vi "Variant To LVType.vi"(8 "error in (no error)":errorcluster, 11 "Variant":variant) -> (0 "error out":errorcluster, 3 "LVType":refnum<class "LVType.lvclass">)   [LabVIEW 2020, in "LVDataTypes.lvlib"]
uses:
  <vilib>/AppBuilder/Engine/WebServiceDescription/LVDataTypes/LVDataTypes.lvlib
  <vilib>/AppBuilder/Engine/WebServiceDescription/LVDataTypes/TypeCode.ctl
  <vilib>/AppBuilder/Engine/WebServiceDescription/LVDataTypes/LVType/LVType.lvclass
  <vilib>/Utility/VariantDataType/Type.ctl
  <vilib>/AppBuilder/Engine/WebServiceDescription/LVDataTypes/LVEnum/LVEnum.lvclass
  e:/builds/penguin/labview/branches/2020/dev/dist/vi.lib/AppBuilder/Engine/WebServiceDescription/LVDataTypes/LVType/LVType.lvclass
  <vilib>/AppBuilder/Engine/WebServiceDescription/LVDataTypes/LVArrayType/LVArrayType.lvclass
  <vilib>/AppBuilder/Engine/WebServiceDescription/LVDataTypes/LVAnalogWaveformType/LVAnalogWaveformType.lvclass
  <vilib>/AppBuilder/Engine/WebServiceDescription/LVDataTypes/LVClusterType/LVClusterType.lvclass
  <vilib>/Utility/VariantDataType/VariantType.lvlib
panel:
  in  "Type Enum":T1
  in  "TypeMap":T2[](array[typedef])=[enum."Undefined", enum."Void", enum."Byte", enum."Word", enum."Long", enum."Quad", enum."Unsigned Byte", enum."Unsigned Word", enum."Unsigned Long", enum."Unsigned Quad", enum."Single", enum."Double", enum."Extended", enum."Complex Single", enum."Complex Double", enum."Complex Extended", enum."Unsigned Byte", enum."Unsigned Word", enum."Unsigned Long", enum."Unsigned Quad", enum."Single", enum."Double", enum."Extended", enum."Complex Single", enum."Complex Double", enum."Complex Extended", enum."Boolean", enum."String", enum."Path", enum."Undefined", enum."Undefined", enum."Array", enum."Cluster", enum."Undefined", enum."Undefined", enum."AnalogWaveform", enum."Time Stamp", enum."DigitalWaveform", enum."Undefined", enum."Undefined", enum."Undefined", enum."Undefined", enum."Undefined", enum."Undefined", enum."Undefined", enum."Undefined"]
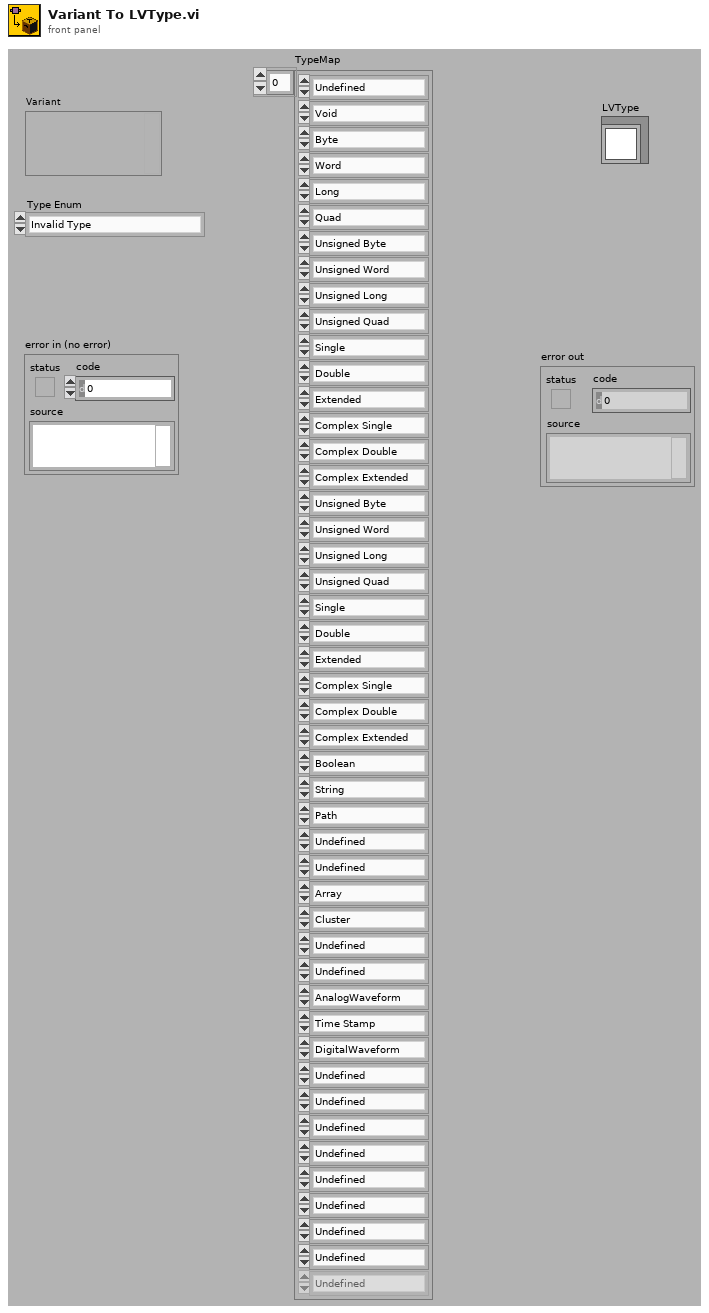
[diagram p1: front panel]
types:
  T1 = typedef "VariantType.lvlib/Type.ctl" = enum8{"Invalid Type", "Void", "I8", "I16", "I32", "I64", "U8", "U16", "U32", "U64", "Single Float", "Double Float", "Extended Float", "Single Complex", "Double Complex", "Extended Complex", "Enum U8", "Enum U16", "Enum U32", "Enum U64", "Single Float With Unit", "Double Float With Unit", "Extended Float With Unit", "Single Complex with Unit", "Double Complex with Unit", "Extended Complex with Unit", "Boolean", "String", "Path", "Picture", "Tag", "Array", "Cluster", "Variant", "LV Variant", "Waveform", "Timestamp", "Digital Waveform", "Digital Data", "ExpressData", "Refnum", "External Data", "VI", "Poly VI", "LabVIEW Class Instance", "Fixed Point"}
  T2 = typedef "LVDataTypes.lvlib/TypeCode.ctl" = enum16{"Undefined", "Byte", "Unsigned Byte", "Word", "Unsigned Word", "Long", "Unsigned Long", "Quad", "Unsigned Quad", "Single", "Double", "Extended", "Enum", "Boolean", "String", "Path", "Array", "Cluster", "AnalogWaveform", "DigitalWaveform", "Time Stamp", "Void", "Complex Single", "Complex Double", "Complex Extended"}
  T3 = typedef "VariantType.lvlib/MemoryInfo.ctl" = cluster{"Type":T4, "Size":u32}
  T4 = typedef "VariantType.lvlib/MemoryType.ctl" = enum16{"Variable", "Fixed", "Bounded"}
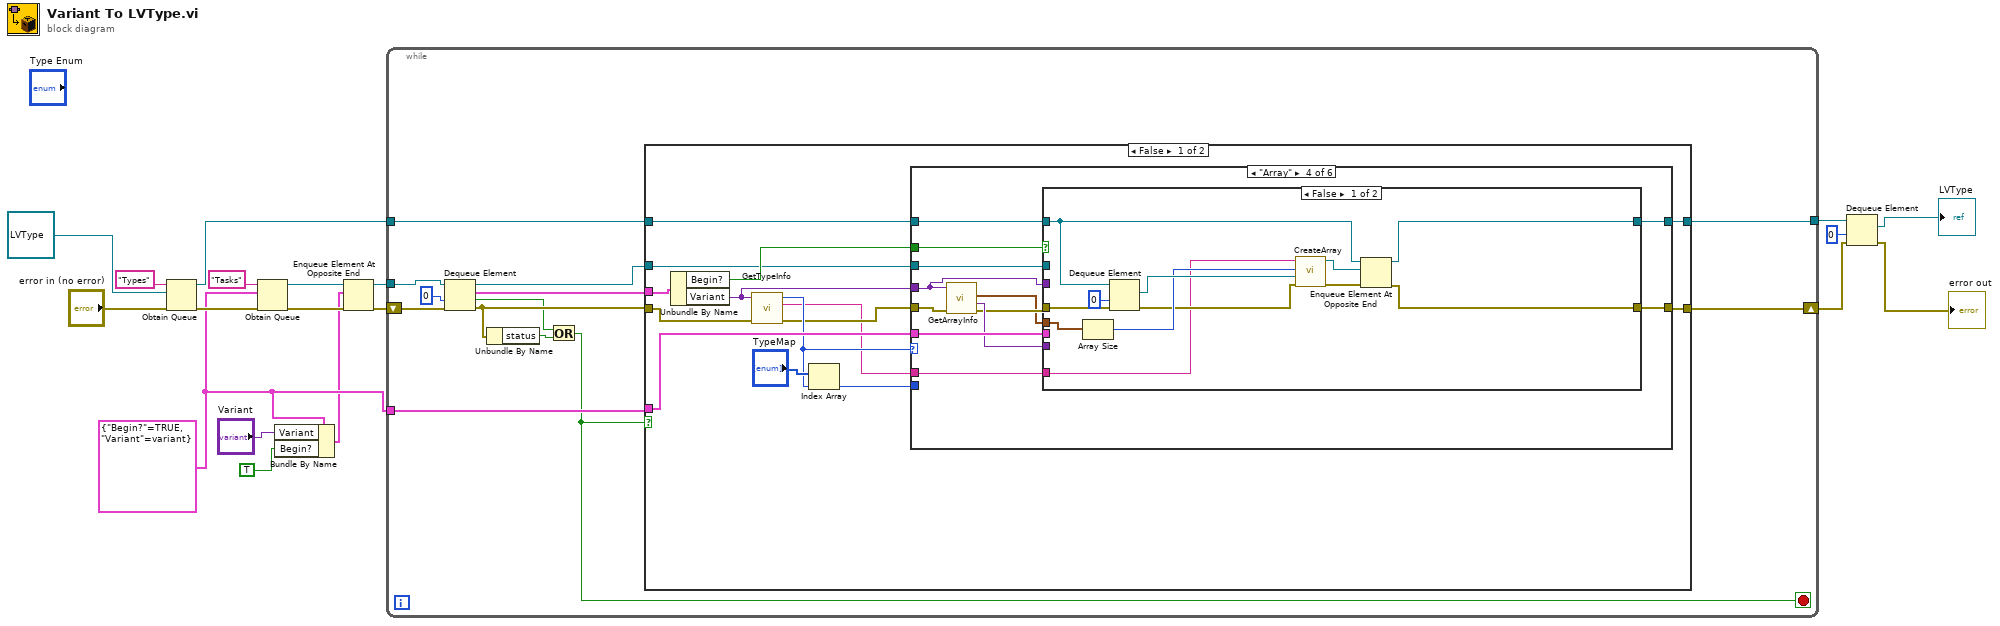
[diagram p0: block diagram]
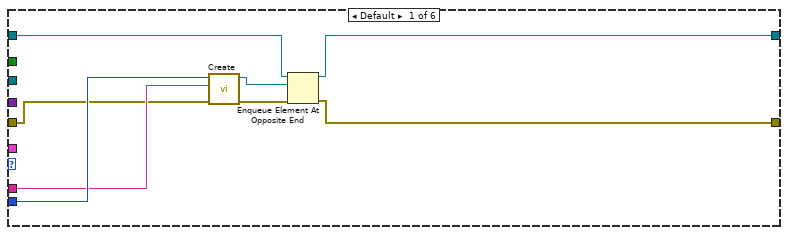
[diagram p2: hidden frame]
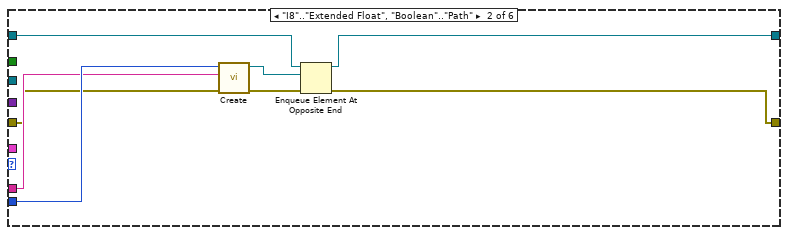
[diagram p3: hidden frame]
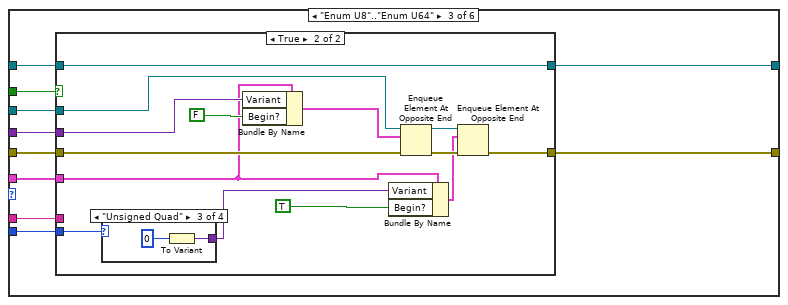
[diagram p4: hidden frame]
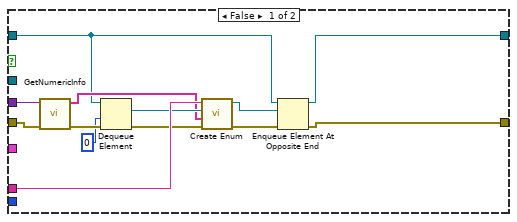
[diagram p5: hidden frame]
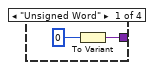
[diagram p6: hidden frame]
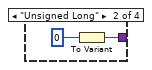
[diagram p7: hidden frame]
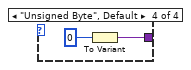
[diagram p8: hidden frame]
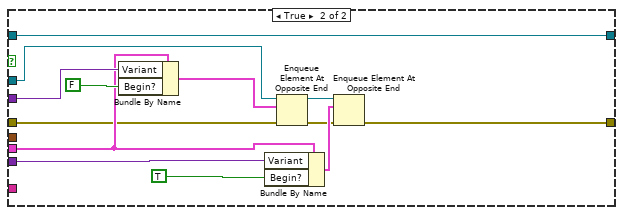
[diagram p9: hidden frame]
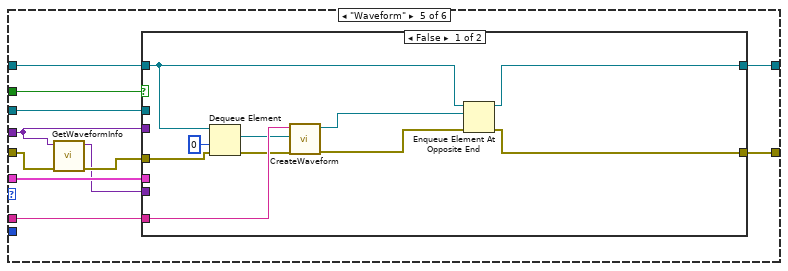
[diagram p10: hidden frame]
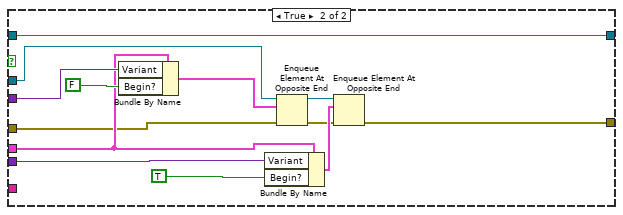
[diagram p11: hidden frame]
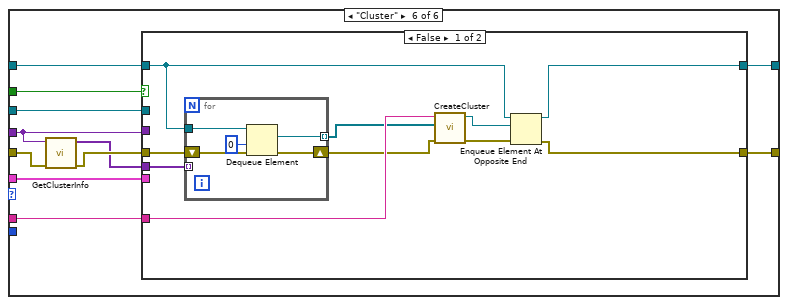
[diagram p12: hidden frame]
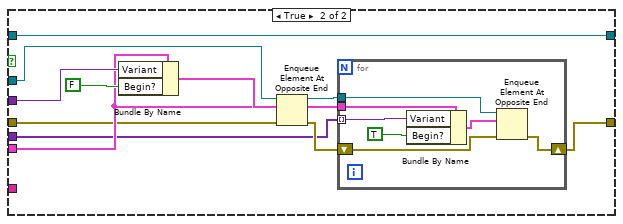
[diagram p13: hidden frame]
diagram:
  w15 = cluster{"Begin?":bool, "Variant":variant} {"Begin?"=TRUE, "Variant"=variant}
  n1 = Obtain Queue(name (unnamed)="Types", element data type=refnum<class "LVType.lvclass"> refnum ("LVDataTypes.lvlib:LVType.lvclass"), error in (no error)="error in (no error)") -> (queue out=w19:refnum<queue>, error out=w18:errorcluster)  [unwired: 2 in, 1 out]
  n2 = Obtain Queue(name (unnamed)="Tasks", element data type=w15, error in (no error)=w18) -> (queue out=w10:refnum<queue>, error out=w12:errorcluster)  [unwired: 2 in, 1 out]
  n3 = Bundle By Name(cluster=w15, "Variant"="Variant", "Begin?"=TRUE) -> (w11:cluster{"Begin?":bool, "Variant":variant})
  n4 = Enqueue Element At Opposite End(queue=w10, element=w11, error in (no error)=w12) -> (queue out=w14:refnum<queue>, error out=w13:errorcluster)  [unwired: 2 out]
  n5 = while {
    tunnel: w14 -> [w32]
    shift-right: [w26] -> w4
    shift-left: w13 -> [w31]
    tunnel: w15 -> [w27]
    tunnel: w19 -> [w25]
    tunnel: [w24] -> w6
    stop <- w20 stop-if-true
    n6 = Dequeue Element(queue=w32, timeout in ms (-1)=0, error in (no error)=w31) -> (queue out=w28:refnum<queue>, element=w29:cluster{"Begin?":bool, "Variant":variant}, timed out?=w21:bool, error out=w23:errorcluster)
    n7 = Unbundle By Name(w23) -> ("status"=w22:bool)
    n8 = Or(x=w21, y=w22) -> (x .or. y?=w20:bool)
    n9 = case shown="False" w20 {
      tunnel: w29 -> [w46 _]
      tunnel: w23 -> [w40 w224]
      tunnel: w28 -> [w44 _]
      tunnel: w27 -> [w43 _]
      tunnel: [w42 w224] -> w26
      tunnel: w25 -> [w41 w223]
      tunnel: [w33 w223] -> w24
      frame False {
        n10 = Unbundle By Name(w46) -> ("Begin?"=w45:bool, "Variant"=w36:variant)
        n11 = call <vilib>:"GetTypeInfo.vi"("error in (no error)"=w40, "Variant"=w36) -> ("error out"=w37:errorcluster, "Name"=w35:string, "Type Enum"=w38:T1)  [unwired: 7 out]
        n12 = Index Array(array="TypeMap", index=w38) -> (element=w34:T2)
        n13 = case shown="\"Array\"" w38 {
          tunnel: w37 -> [w52 w60 w67 w114 w147 w181]
          tunnel: w45 -> [_ _ w69 w119 w155 w189]
          tunnel: w44 -> [_ _ w70 w118 w154 w188]
          tunnel: w43 -> [_ _ w66 w117 w153 w187]
          tunnel: [w47 w58 w63 w116 w152 w186] -> w42
          tunnel: w41 -> [w50 w57 w72 w115 w151 w185]
          tunnel: w36 -> [_ _ w68 w113 w148 w182]
          tunnel: w35 -> [w53 w61 w64 w109 w150 w184]
          tunnel: w34 -> [w54 w62 w65 _ _ _]
          tunnel: [w48 w55 w71 w108 w149 w183] -> w33
          frame Default {
            n14 = call <vilib>:"Create.vi"("error in (no error)"=w52, "ID"=w53, "Type"=w54) -> ("error out"=w51:errorcluster, "LVType out"=w49:refnum<class "LVType.lvclass">)  [unwired: 7 out]
            n15 = Enqueue Element At Opposite End(queue=w50, element=w49, error in (no error)=w51) -> (queue out=w48:refnum<queue>, error out=w47:errorcluster)  [unwired: 2 out]
          }
          frame "I8".."Extended Float", "Boolean".."Path" {
            n16 = call <vilib>:"Create.vi"("error in (no error)"=w60, "ID"=w61, "Type"=w62) -> ("error out"=w59:errorcluster, "LVType out"=w56:refnum<class "LVType.lvclass">)  [unwired: 7 out]
            n17 = Enqueue Element At Opposite End(queue=w57, element=w56, error in (no error)=w59) -> (queue out=w55:refnum<queue>, error out=w58:errorcluster)  [unwired: 2 out]
          }
          frame "Enum U8".."Enum U64" {
            n18 = case shown="True" w69 {
              tunnel: w72 -> [w77 w93]
              tunnel: [w73 w93] -> w71
              tunnel: w70 -> [_ w92]
              tunnel: w68 -> [w85 w91]
              tunnel: w67 -> [w84 w90]
              tunnel: w66 -> [_ w89]
              tunnel: w65 -> [_ w88]
              tunnel: w64 -> [w81 _]
              tunnel: [w74 w86] -> w63
              frame False {
                n19 = call <vilib>:"GetNumericInfo.vi"("error in (no error)"=w84, "Variant"=w85) -> ("error out"=w83:errorcluster, "EnumNames"=w79:string[])  [unwired: 8 out]
                n20 = Dequeue Element(queue=w77, timeout in ms (-1)=0, error in (no error)=w83) -> (element=w80:refnum<class "LVType.lvclass">, error out=w78:errorcluster)  [unwired: 2 out]
                n21 = call <vilib>:"Create Enum.vi"("error in (no error)"=w78, "Choices"=w79, "BaseType"=w80, "ID"=w81) -> ("error out"=w76:errorcluster, "LVEnum out"=w75:refnum<class "LVEnum.lvclass">)  [unwired: 6 out]
                n22 = Enqueue Element At Opposite End(queue=w77, element=w75, error in (no error)=w76) -> (queue out=w73:refnum<queue>, error out=w74:errorcluster)  [unwired: 2 out]
              }
              frame True {
                n23 = case shown="\"Unsigned Quad\"" w88 {
                  tunnel: [w100 w102 w104 w106] -> w87
                  frame "Unsigned Word" {
                    n24 = To Variant(anything=u16 0) -> (Variant=w100:variant)
                  }
                  frame "Unsigned Long" {
                    n25 = To Variant(anything=u32 0) -> (Variant=w102:variant)
                  }
                  frame "Unsigned Quad" {
                    n26 = To Variant(anything=u64 0) -> (Variant=w104:variant)
                  }
                  frame "Unsigned Byte", Default {
                    n27 = To Variant(anything=u8 0) -> (Variant=w106:variant)
                  }
                }
                n28 = Bundle By Name(cluster=w89, "Variant"=w91, "Begin?"=FALSE) -> (w95:cluster{"Begin?":bool, "Variant":variant})
                n29 = Bundle By Name(cluster=w89, "Variant"=w87, "Begin?"=TRUE) -> (w97:cluster{"Begin?":bool, "Variant":variant})
                n30 = Enqueue Element At Opposite End(queue=w92, element=w95, error in (no error)=w90) -> (queue out=w99:refnum<queue>, error out=w98:errorcluster)  [unwired: 2 out]
                n31 = Enqueue Element At Opposite End(queue=w99, element=w97, error in (no error)=w98) -> (error out=w86:errorcluster)  [unwired: 3 out]
              }
            }
          }
          frame "Array" {
            n32 = call <vilib>:"GetArrayInfo.vi"("error in (no error)"=w114, "Variant"=w113) -> ("error out"=w111:errorcluster, "ArrayElement"=w112:variant, "Array Lengths"=w110:T3[])  [unwired: 7 out]
            n33 = case shown="False" w119 {
              tunnel: w113 -> [_ w141]
              tunnel: w118 -> [_ w142]
              tunnel: w117 -> [_ w138]
              tunnel: [w122 w135] -> w116
              tunnel: w115 -> [w124 w132]
              tunnel: w111 -> [w131 w133]
              tunnel: w112 -> [_ w134]
              tunnel: w110 -> [w128 _]
              tunnel: w109 -> [w125 _]
              tunnel: [w121 w132] -> w108
              frame False {
                n34 = Array Size(array=w128) -> (size(s)=w127:i32)
                n35 = Dequeue Element(queue=w124, timeout in ms (-1)=0, error in (no error)=w131) -> (element=w129:refnum<class "LVType.lvclass">, error out=w126:errorcluster)  [unwired: 2 out]
                n36 = call <vilib>:"CreateArray.vi"("error in (no error)"=w126, "ChildType"=w129, "Dimension"=w127, "ID"=w125) -> ("error out"=w123:errorcluster, "LVArrayType out"=w120:refnum<class "LVArrayType.lvclass">)  [unwired: 6 out]
                n37 = Enqueue Element At Opposite End(queue=w124, element=w120, error in (no error)=w123) -> (queue out=w121:refnum<queue>, error out=w122:errorcluster)  [unwired: 2 out]
              }
              frame True {
                n38 = Bundle By Name(cluster=w138, "Variant"=w141, "Begin?"=FALSE) -> (w143:cluster{"Begin?":bool, "Variant":variant})
                n39 = Bundle By Name(cluster=w138, "Variant"=w134, "Begin?"=TRUE) -> (w139:cluster{"Begin?":bool, "Variant":variant})
                n40 = Enqueue Element At Opposite End(queue=w142, element=w143, error in (no error)=w133) -> (queue out=w136:refnum<queue>, error out=w137:errorcluster)  [unwired: 2 out]
                n41 = Enqueue Element At Opposite End(queue=w136, element=w139, error in (no error)=w137) -> (error out=w135:errorcluster)  [unwired: 3 out]
              }
            }
          }
          frame "Waveform" {
            n42 = call <vilib>:"GetWaveformInfo.vi"("error in (no error)"=w147, "Variant"=w148) -> ("error out"=w146:errorcluster, "YArrayType"=w145:variant)  [unwired: 8 out]
            n43 = case shown="False" w155 {
              tunnel: w148 -> [_ w175]
              tunnel: w154 -> [_ w176]
              tunnel: w153 -> [_ w172]
              tunnel: [w163 w169] -> w152
              tunnel: w151 -> [w164 w167]
              tunnel: w145 -> [_ w168]
              tunnel: w150 -> [w161 _]
              tunnel: [w162 w167] -> w149
              tunnel: w146 -> [w156 w166]
              frame False {
                n44 = Dequeue Element(queue=w164, timeout in ms (-1)=0, error in (no error)=w156) -> (element=w159:refnum<class "LVType.lvclass">, error out=w160:errorcluster)  [unwired: 2 out]
                n45 = call <vilib>:"CreateWaveform.vi"("error in (no error)"=w160, "YArrayType"=w159, "ID"=w161) -> ("error out"=w158:errorcluster, "LVAnalogWaveformType out"=w157:refnum<class "LVAnalogWaveformType.lvclass">)  [unwired: 7 out]
                n46 = Enqueue Element At Opposite End(queue=w164, element=w157, error in (no error)=w158) -> (queue out=w162:refnum<queue>, error out=w163:errorcluster)  [unwired: 2 out]
              }
              frame True {
                n47 = Bundle By Name(cluster=w172, "Variant"=w175, "Begin?"=FALSE) -> (w177:cluster{"Begin?":bool, "Variant":variant})
                n48 = Bundle By Name(cluster=w172, "Variant"=w168, "Begin?"=TRUE) -> (w173:cluster{"Begin?":bool, "Variant":variant})
                n49 = Enqueue Element At Opposite End(queue=w176, element=w177, error in (no error)=w166) -> (queue out=w170:refnum<queue>, error out=w171:errorcluster)  [unwired: 2 out]
                n50 = Enqueue Element At Opposite End(queue=w170, element=w173, error in (no error)=w171) -> (error out=w169:errorcluster)  [unwired: 3 out]
              }
            }
          }
          frame "Cluster" {
            n51 = call <vilib>:"GetClusterInfo.vi"("error in (no error)"=w181, "Variant"=w182) -> ("error out"=w180:errorcluster, "Cluster Elements"=w179:variant[])  [unwired: 8 out]
            n52 = case shown="False" w189 {
              tunnel: w182 -> [_ w212]
              tunnel: w188 -> [_ w213]
              tunnel: w187 -> [_ w211]
              tunnel: [w191 w206] -> w186
              tunnel: w185 -> [w192 w209]
              tunnel: w180 -> [w199 w210]
              tunnel: w184 -> [w197 _]
              tunnel: [w190 w209] -> w183
              tunnel: w179 -> [w198 w205]
              frame False {
                n53 = for {
                  tunnel: w192 -> [w202]
                  tunnel: w198 -> [_] mode=indexing
                  tunnel: [w201] -> w196 mode=indexing
                  shift-right: [w200] -> w195
                  shift-left: w199 -> [w204]
                  n54 = Dequeue Element(queue=w202, timeout in ms (-1)=0, error in (no error)=w204) -> (element=w201:refnum<class "LVType.lvclass">, error out=w200:errorcluster)  [unwired: 2 out]
                }
                n55 = call <vilib>:"CreateCluster.vi"("error in (no error)"=w195, "ChildTypes"=w196, "ID"=w197) -> ("error out"=w194:errorcluster, "LVClusterType out"=w193:refnum<class "LVClusterType.lvclass">)  [unwired: 7 out]
                n56 = Enqueue Element At Opposite End(queue=w192, element=w193, error in (no error)=w194) -> (queue out=w190:refnum<queue>, error out=w191:errorcluster)  [unwired: 2 out]
              }
              frame True {
                n57 = Bundle By Name(cluster=w211, "Variant"=w212, "Begin?"=FALSE) -> (w214:cluster{"Begin?":bool, "Variant":variant})
                n58 = Enqueue Element At Opposite End(queue=w213, element=w214, error in (no error)=w210) -> (queue out=w207:refnum<queue>, error out=w208:errorcluster)  [unwired: 2 out]
                n59 = for {
                  tunnel: w211 -> [w220]
                  shift-right: [w218] -> w206
                  shift-left: w208 -> [w219]
                  tunnel: w207 -> [w217]
                  tunnel: w205 -> [w216] mode=indexing
                  n60 = Bundle By Name(cluster=w220, "Variant"=w216, "Begin?"=TRUE) -> (w221:cluster{"Begin?":bool, "Variant":variant})
                  n61 = Enqueue Element At Opposite End(queue=w217, element=w221, error in (no error)=w219) -> (error out=w218:errorcluster)  [unwired: 3 out]
                }
              }
            }
          }
        }
      }
      frame True {
      }
    }
  }
  n62 = Dequeue Element(queue=w6, timeout in ms (-1)=0, error in (no error)=w4) -> (element=→"LVType":refnum<class "LVType.lvclass">, error out=→"error out":errorcluster)  [unwired: 2 out]
